vi "set keypair ocsp mem.vi"(7 "staple":string, 8 "error in":errorcluster, 9 "key":string, 10 "cert":string, 11 "lvlibretls configurable context in":refnum<class "lvlibretls configurable context.lvclass">) -> (0 "error out":errorcluster, 3 "lvlibretls configurable context out":refnum<class "lvlibretls configurable context.lvclass">)   [LabVIEW 2016, in "lvlibretls configurable context.lvclass"]
uses:
  lvlibretls configurable context.lvclass
  lvlibretls configurable context.lvclass/lvlibretls configurable context.ctl
  lv tls dll.lvlib
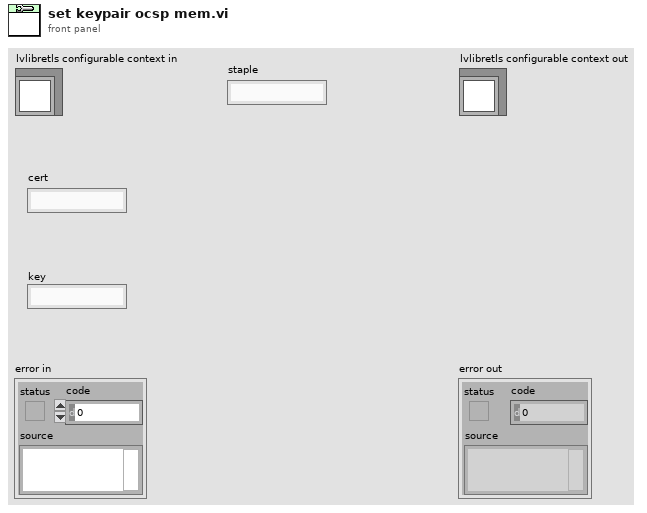
[diagram p1: front panel]
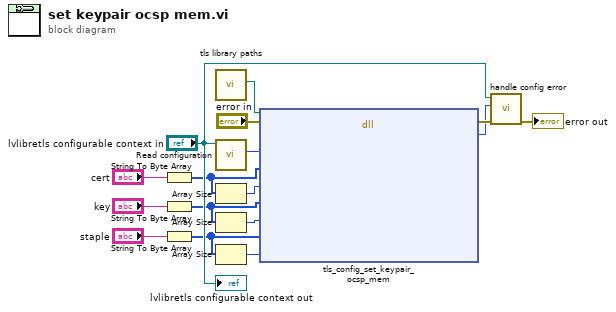
[diagram p0: block diagram]
diagram:
  n1 = String To Byte Array(string="cert") -> (unsigned byte array=w7:u8[])
  n2 = String To Byte Array(string="key") -> (unsigned byte array=w4:u8[])
  n3 = String To Byte Array(string="staple") -> (unsigned byte array=w1:u8[])
  n4 = call "tls library paths.vi"() -> ("libtls"=w16:path)  [unwired: 8 in, 3 out]
  n5 = call "Read configuration.vi"("lvlibretls configurable context in"="lvlibretls configurable context in") -> ("configuration"=w15:u64)  [unwired: 10 in]
  n6 = Array Size(array=w7) -> (size(s)=w6:i32)
  n7 = Array Size(array=w4) -> (size(s)=w5:i32)
  n8 = Array Size(array=w1) -> (size(s)=w2:i32)
  n9 = dll-call lib="C:/Users/IEUser/Desktop/tlssimple/libtls-15.dll" fn="tls_config_set_keypair_ocsp_mem"(path in=w16, error in="error in", "config"=w15, "certfile"=w7, "certlen"=w6, "keyfile"=w4, "keylen"=w5, "staplefile"=w1, "staplelen"=w2) -> (error out=w14:errorcluster, "return"=w13:i32)  [unwired: 8 in, 1 out]
  n10 = call "handle config error.vi"("error in"=w14, "return"=w13, "lvlibretls configurable context in"="lvlibretls configurable context in") -> ("error out"=→"error out":errorcluster)  [unwired: 8 in]
  "lvlibretls configurable context out" <- "lvlibretls configurable context in"
